vi "Get Data I16_32.vi"(8 "error in (no error)":errorcluster, 11 "Ni-Scope Digitizer in":refnum<class "Ni-Scope Digitizer.lvclass">) -> (0 "error out":errorcluster, 1 "I32 data out":i32[][](array[numeric]), 2 "I16 data out":i16[][](array[numeric]), 3 "Ni-Scope Digitizer out":refnum<class "Ni-Scope Digitizer.lvclass">, 4 "Finished":bool, 5 "Current read position":i32)   [LabVIEW 2016, in "Ni-Scope Digitizer.lvclass"]
uses:
  Ni-Scope Digitizer.lvclass
  C:/github/NHMFL_Core/Libraries/Instruments/Pulse Driver/Pulse Driver.lvclass
  Ni-Scope Digitizer.lvclass/Ni-Scope Digitizer.ctl
  Instruments/Pulse Driver/Pulse Driver.lvclass/Pulse Driver.ctl
  Instruments/Pulse Driver/Read Samples per channel.vi
  Instruments/Pulse Driver/Read Current read position.vi
  Instruments/Pulse Driver/Read Samples per read.vi
  Instruments/Pulse Driver/Read Binary sample width.vi
  Read Fetch Relative To.vi
  Write instrument handle.vi
  <instrlib>/niScope/Acquire/Fetch/niScope Multi Fetch Binary 16.vi
  <instrlib>/niScope/Acquire/Fetch/niScope Multi Fetch Binary 32.vi
panel:
  out "Horizontal:Reference Position":dbl
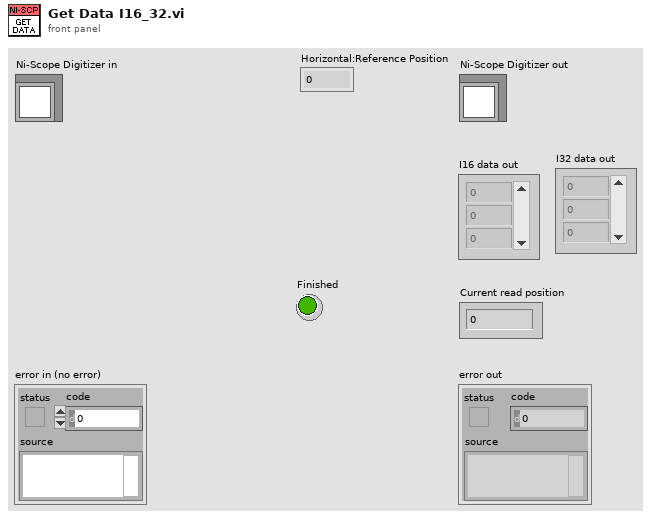
[diagram p1: front panel]
types:
  T1 = typedef "Pusle Driver Configuration.ctl" = cluster{"Pre-trigger duration":dbl, "Post-trigger duration":dbl, "Rate":dbl, "Ranges":dbl[], "Re-name channels":string[], "Active channels":string, "External clock":bool}
  T2 = cluster{"actualSamples":i32, "absoluteInitialX":dbl, "relativeInitialX":dbl, "xIncrement":dbl, "offset":dbl, "gain":dbl, "reserved1":dbl, "reserved2":dbl}[]
  T3 = cluster{"actualSamples":i32, "absoluteInitialX":dbl, "relativeInitialX":dbl, "xIncrement":dbl, "offset":dbl, "gain":dbl, "reserved1":dbl, "reserved2":dbl}
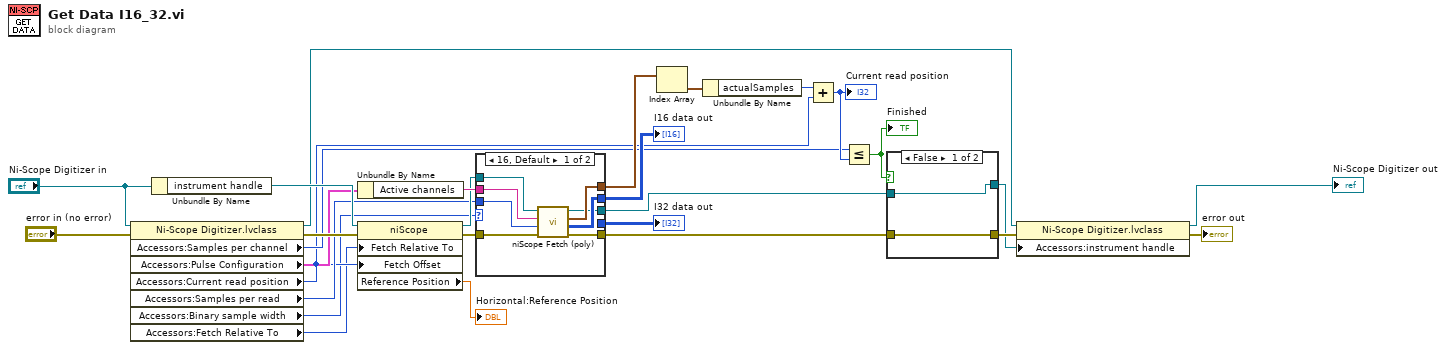
[diagram p0: block diagram]
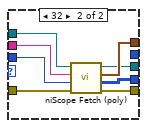
[diagram p2: hidden frame]
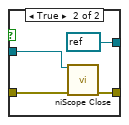
[diagram p3: hidden frame]
diagram:
  n1 = property class="Ni-Scope Digitizer.lvclass"(reference="Ni-Scope Digitizer in", error in="error in (no error)") -> (reference out=w3:refnum<class "Ni-Scope Digitizer.lvclass">, error out=w23:errorcluster, "Accessors:Samples per channel"=w13:i32, "Accessors:Pulse Configuration"=w12:T1, "Accessors:Current read position"=w9:i32, "Accessors:Samples per read"=w11:i32, "Accessors:Binary sample width"=w7:i32, "Accessors:Fetch Relative To"=w5:i32)
  n2 = Unbundle By Name("Ni-Scope Digitizer in") -> ("instrument handle"=w26:refnum<k15>)
  n3 = Unbundle By Name(w12) -> ("Active channels"=w28:string)
  n4 = property class="niScope"(reference=w26, error in=w23, "Fetch Relative To"=w5, "Fetch Offset"=w9) -> (reference out=w25:refnum<k15>, error out=w24:errorcluster, "Reference Position"=→"Horizontal:Reference Position":dbl)
  n5 = case shown="16, Default" w7 {
    tunnel: w28 -> [w36 w44]
    tunnel: w25 -> [w35 w43]
    tunnel: w24 -> [w34 w42]
    tunnel: [w33 w41] -> w21
    tunnel: [w32 _] -> w20
    tunnel: [w31 w40] -> w19
    tunnel: [w30 w39] -> w15
    tunnel: w11 -> [w29 w38]
    tunnel: [_ w37] -> w6
    frame 16, Default {
      n6 = call-poly <instrlib>:"niScope Fetch (poly).vi"("error in"=w34, "numSamples"=w29, "channels"=w36, "instrument handle"=w35) -> ("error out"=w33:errorcluster, "wfm"=w32:i16[][], "wfm info"=w31:T2, "instrument handle out"=w30:refnum<k15>)  [unwired: 4 in]
    }
    frame 32 {
      n7 = call-poly <instrlib>:"niScope Fetch (poly).vi"("error in"=w42, "numSamples"=w38, "channels"=w44, "instrument handle"=w43) -> ("error out"=w41:errorcluster, "wfm"=w37:i32[][], "wfm info"=w40:T2, "instrument handle out"=w39:refnum<k15>)  [unwired: 4 in]
    }
  }
  "I16 data out" <- w20
  "I32 data out" <- w6
  n8 = Index Array(array=w19) -> (element=w18:T3)  [unwired: 1 in]
  n9 = Unbundle By Name(w18) -> ("actualSamples"=w17:i32)
  n10 = Add(x=w17, y=w9) -> (x+y=w16:i32)
  "Current read position" <- w16
  n11 = Less Or Equal?(x=w13, y=w16) -> (x <= y?=w10:bool)
  "Finished" <- w10
  n12 = case shown="False" w10 {
    tunnel: [w46 w50] -> w14
    tunnel: w15 -> [w45 w49]
    tunnel: w21 -> [w46 w48]
    tunnel: [w45 refnum<k15> refnum ("instrument handle out")] -> w1
    frame False {
    }
    frame True {
      n13 = call <instrlib>:"niScope Close.vi"("instrument handle"=w49, "error in"=w48) -> ("error out"=w50:errorcluster)  [unwired: 13 out]
    }
  }
  n14 = property class="Ni-Scope Digitizer.lvclass"(reference=w3, error in=w14, "Accessors:instrument handle"=w1) -> (reference out=→"Ni-Scope Digitizer out":refnum<class "Ni-Scope Digitizer.lvclass">, error out=→"error out":errorcluster)
